vi "Handle setAllData.vi"(8 "error in (no error)":errorcluster, 10 "AllData":variant, 11 "instrument.Cryostation in":refnum<class "instrument.Cryostation.lvclass">) -> (0 "error out":errorcluster, 3 "instrument.Cryostation out":refnum<class "instrument.Cryostation.lvclass">)   [LabVIEW 2019, in "instrument.Cryostation.lvclass"]
doc: "Override to handle incoming \"setAllData\" command for <b>your</b> Instrument"
uses:
  instrument.Cryostation.lvclass
  instrument.Cryostation.lvclass/instrument.Cryostation.ctl
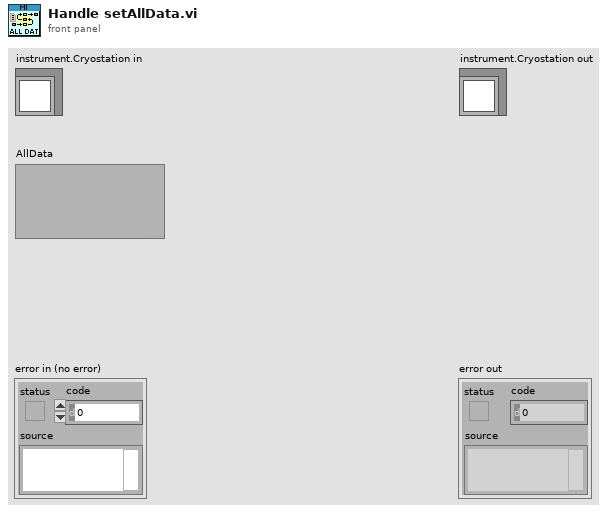
[diagram p1: front panel]
types:
  T1 = typedef "instrument.Cryostation.lvclass/Cryostation.getAll--cluster.ctl" = cluster{"Chamber Pressure (mTorr)":dbl, "Compressor Return Pressure (MPa)":dbl, "Compressor Supply Pressure (MPa)":dbl, "Compressor Speed (Hz)":dbl, "Cold Head Speed (Hz)":dbl, "Platform Heater Power (W)":dbl, "Platform Stability (K)":dbl, "Platform Temperature (K)":dbl, "Stage 1 Heater Power (W)":dbl, "Stage 1 Temperature (K)":dbl, "Stage 2 Heater Power (W)":dbl, "Stage 2 Temperature (K)":dbl, "Sample Stability (K)":dbl, "Sample Temperature (K)":dbl, "Temperature Set Point (K)":dbl, "User Stability (K)":dbl, "User Temperature (K)":dbl, "User Temperature Set Point (K)":dbl, "Alarm State":string, "Compressor Run State":string, "Case Valve State":string, "Idle State":string, "Nitrogen State":string, "Vent Valve State":string}
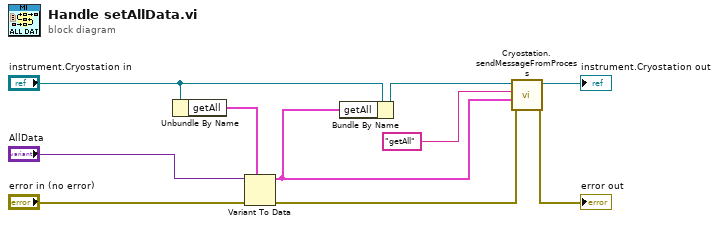
[diagram p0: block diagram]
diagram:
  n1 = Unbundle By Name("instrument.Cryostation in") -> ("getAll"=w7:T1)
  n2 = Variant To Data(error in="error in (no error)", type=w7, Variant="AllData") -> (data=w2:T1, error out=w5:errorcluster)
  n3 = Bundle By Name(cluster="instrument.Cryostation in", "getAll"=w2) -> (w6:refnum<class "instrument.Cryostation.lvclass">)
  n4 = call "Cryostation.sendMessageFromProcess.vi"("error in (no error)"=w5, "Data"=w2, "Command"="getAll", "instrument.Cryostation"=w6) -> ("error out"=→"error out":errorcluster, "instrument.Cryostation out"=→"instrument.Cryostation out":refnum<class "instrument.Cryostation.lvclass">)  [unwired: 6 in]
